vi "Exemple_Metrics_Pairwise_Linear_Kernel.vi"() -> ()   [LabVIEW 2020]
uses:
  Objet/6 - Datasets Transformation/6.8 - Pairwise metrics, Affinities and Kernels/Linear_kernel/Linear_kernel.vi
panel:
  in  "linear_kernel":cluster{"dense_output":bool}={"dense_output"=TRUE}
  in  "error in":errorcluster caption="entrée d'erreur"
  in  "Y":string[][](array[string])
  in  "X":string[][](array[string])=[["0", "1"], ["1", "0"], ["2", "8"], ["7", "3"]]
  out "Data":T1
  out "error out":errorcluster caption="sortie d'erreur"
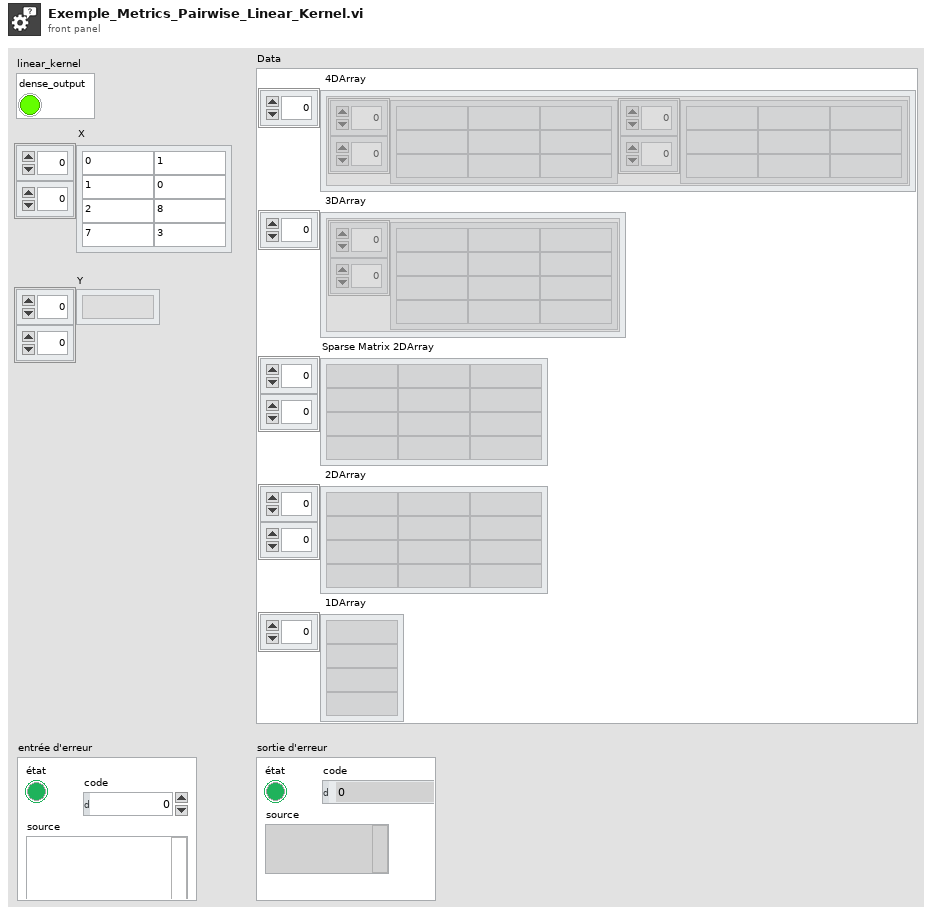
[diagram p1: front panel]
types:
  T1 = cluster{" 4DArray":cluster{"1":string[][], "2":string[][]}[], " 3DArray":cluster{"Tableau":string[][]}[], "Sparse Matrix 2DArray":string[][], " 2DArray":string[][], " 1DArray":string[]}
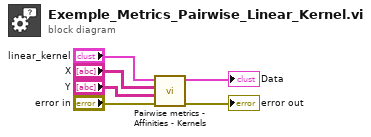
[diagram p0: block diagram]
diagram:
  n1 = call-poly "Pairwise metrics - Affinities - Kernels.vi"("error in"="error in", "Y"="Y", "X"="X", "linear_kernel"="linear_kernel") -> ("error out"=→"error out":errorcluster, "Data"=→"Data":T1)  [unwired: 6 in]
